vi "LVClass_CameraSet Set Parameter IntValue.vi"(0 "CameraSet.lvclass":refnum<class "CameraSet.lvclass">, 5 "parameter_name":string, 7 "Value":i32, 11 "error in (no error)":errorcluster) -> (4 "CameraSet.lvclass":refnum<class "CameraSet.lvclass">, 15 "error out":errorcluster)   [LabVIEW 2020, in "CameraSet.lvclass"]
doc: "Camera parameter value setter for parameter of type integer.\n\n<B>camera_setIn</B> : CameraSet object.\n<B>camera_setOut</B> : CameraSet object.\n<B>parameter_name</B> : Parameter name.\n<B>value</B> : Parameter value."
uses:
  CameraSet.lvclass
  CameraSet.lvclass/CameraSet.ctl
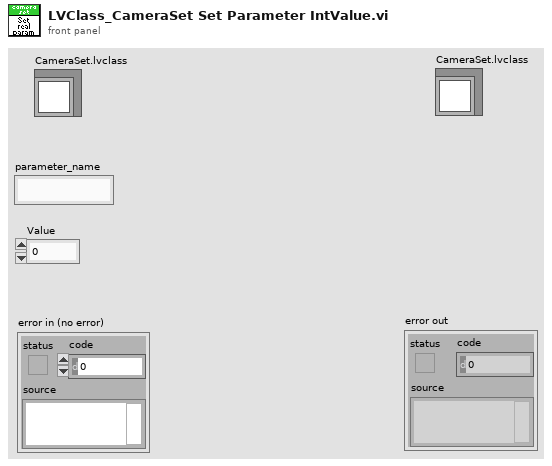
[diagram p1: front panel]
types:
  T1 = typedef "ClassID.ctl" = i64
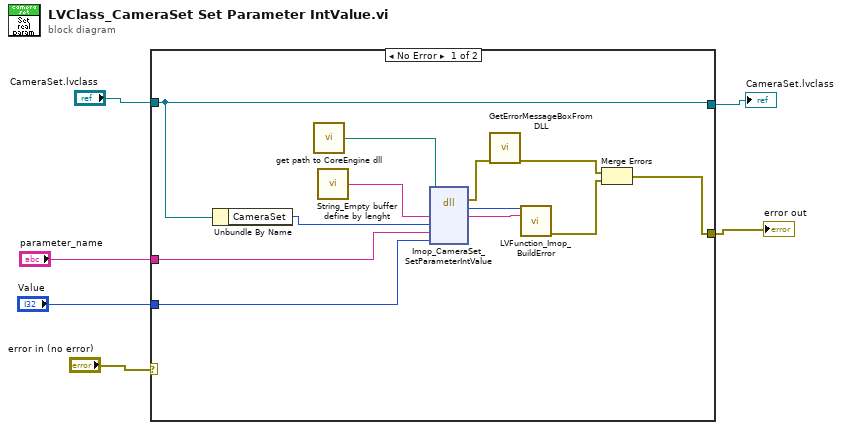
[diagram p0: block diagram]
diagram:
  n1 = case shown="No Error" "error in (no error)" {
    selector: "error in (no error)" -> [_ w19]
    tunnel: "CameraSet.lvclass" -> [w13 w20]
    tunnel: [w13 w20] -> w4
    tunnel: [w9 w19] -> w3
    tunnel: "parameter_name" -> [w8 _]
    tunnel: "Value" -> [w7 _]
    frame No Error {
      n2 = Unbundle By Name(w13) -> ("CameraSet"=w12:T1)
      n3 = call "get path to CoreEngine dll.vi"() -> ("path to wavekit library"=w15:path)  [unwired: 14 in, 1 out]
      n4 = call "String_Empty buffer define by lenght.vi"() -> ("Empty buffer"=w16:string)  [unwired: 1 in]
      n5 = dll-call lib="D:/2_trunk/Soft_haso/ImOpCoreEngine4_LV2011/DLLs/ImopEngine4_vc100.dll" fn="Imop_CameraSet_SetParameterIntValue"(path in=w15, "message"=w16, "objet"=w12, "parameter_name"=w8, "value"=w7) -> (error out=w14:errorcluster, "return type"=w18:i32, "message"=w17:string)  [unwired: 5 in, 1 out]
      n6 = call "GetErrorMessageBoxFromDLL.vi"("error IN"=w14) -> ("error OUT"=w10:errorcluster)  [unwired: 10 in]
      n7 = call "LVFunction_Imop_BuildError.vi"("code"=w18, "String to Prepend to source (\"\")"=w17) -> ("error out"=w11:errorcluster)  [unwired: 13 in]
      n8 = Merge Errors(w10, w11) -> (w9:errorcluster)
    }
    frame Error {
    }
  }
  "CameraSet.lvclass" <- w4
  "error out" <- w3
